vi "Motion Compensation Metrics.vi"() -> ()   [LabVIEW 2011]
uses:
  <vilib>/vision/NI_Vision_Development_Module.lvlib
panel:
  out "Waveform Chart 6":sgl(graph)
  out "Waveform Chart 5":sgl(graph)
  out "Waveform Chart 4":sgl(graph)
  out "Waveform Chart 3":sgl(graph)
  out "Waveform Chart 2":sgl[](graph)
  out "Waveform Chart":sgl[](graph)
  # "Orginal"
  # "Stabilized"
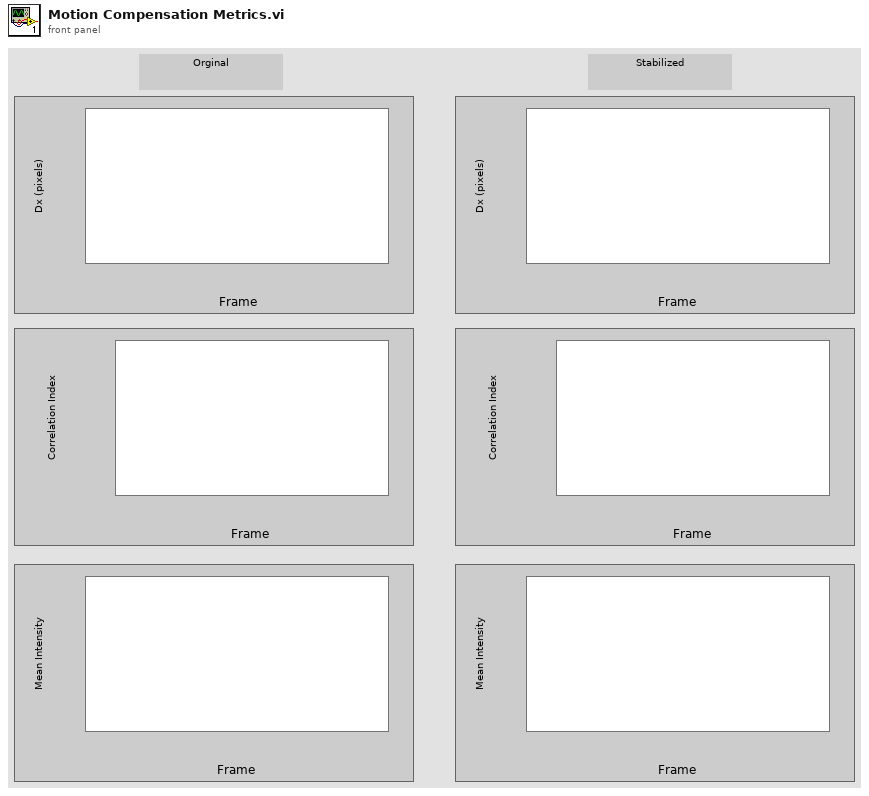
[diagram p1: front panel]
types:
  T1 = typedef "AviRefnum.ctl" = refnum<k1>
  T2 = typedef "IMAQ Image.ctl" = refnum<image>
  T3 = typedef "IMAQ Rectangle" = cluster{"Left":i32, "Top":i32, "Right":i32, "Bottom":i32, "Rotation":dbl}
  T4 = typedef "ROI Descriptor" = cluster{"Global Rectangle":i32[], "Contours":cluster{"ID":enum32{"External", "Internal"}, "Type":u32, "Coordinates":i32[]}[]}
  T5 = cluster{"Mean Intensity":sgl, "Standard  Deviation":sgl, "Minimum Intensity":sgl, "Maximum Intensity":sgl}
  T6 = cluster{"Position":cluster{"x":sgl, "y":sgl}, "Angle":sgl, "Scale":sgl, "Score":sgl, "Bounding Box":cluster{"x":sgl, "y":sgl}[]}[]
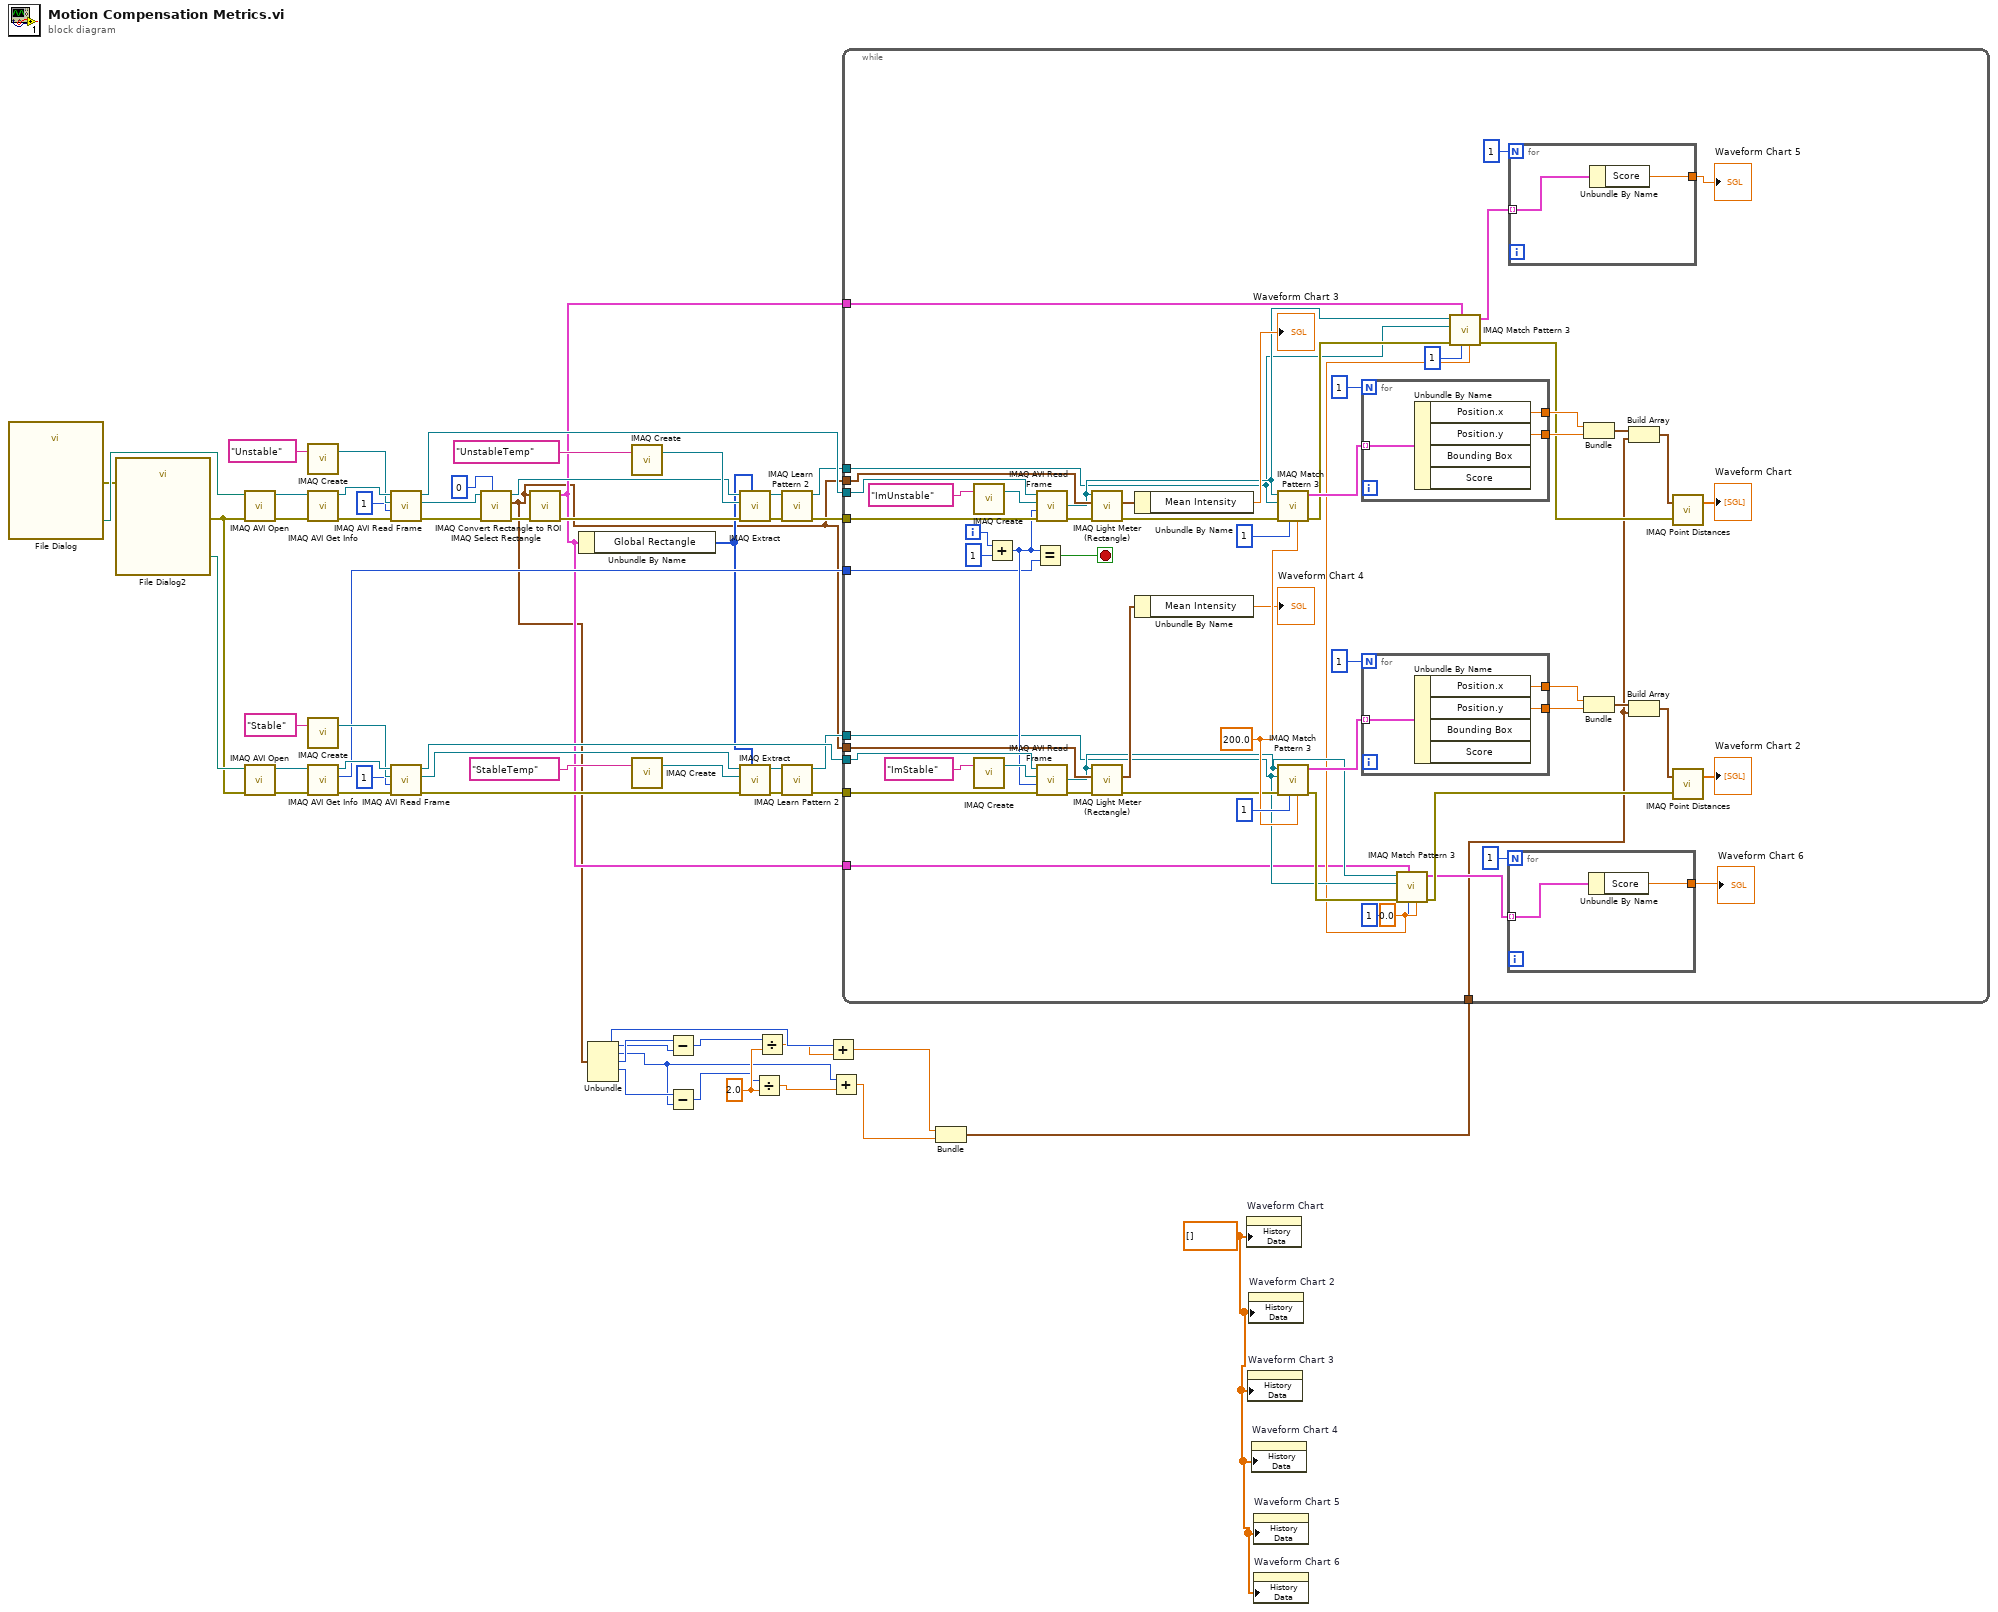
[diagram p0: block diagram]
diagram:
  w11 = 2.0 ("y")
  w14 = sgl[] [] ("History Data")
  n1 = call "File Dialog"() -> ("selected path"=w53:path, "error out"=w45:errorcluster)  [unwired: 12 in, 2 out]
  n2 = call "File Dialog2"("error in"=w45) -> ("selected path"=w52:path, "error out"=w44:errorcluster)  [unwired: 11 in, 2 out]
  n3 = call "IMAQ AVI Open"("error in (no error)"=w44, "AVI Path"=w53) -> ("error out"=w56:errorcluster, "Avi Refnum"=w51:T1)  [unwired: 8 in]
  n4 = call "IMAQ AVI Open"("error in (no error)"=w44, "AVI Path"=w52) -> ("error out"=w57:errorcluster, "Avi Refnum"=w50:T1)  [unwired: 8 in]
  n5 = call "IMAQ Create"("Image Name"="Unstable") -> ("New Image"=w46:T2)  [unwired: 4 in, 1 out]
  n6 = call "IMAQ AVI Get Info"("error in (no error)"=w56, "Avi Refnum"=w51) -> ("error out"=w55:errorcluster, "Avi Refnum (duplicate)"=w49:T1)  [unwired: 5 in, 3 out]
  n7 = call "IMAQ Create"("Image Name"="Stable") -> ("New Image"=w47:T2)  [unwired: 4 in, 1 out]
  n8 = call "IMAQ AVI Get Info"("error in (no error)"=w57, "Avi Refnum"=w50) -> ("error out"=w54:errorcluster, "Number of Frames"=w32:u32, "Avi Refnum (duplicate)"=w48:T1)  [unwired: 5 in, 2 out]
  n9 = call "IMAQ AVI Read Frame"("error in (no error)"=w55, "Frame Number"=u32 1, "Image"=w46, "Avi Refnum"=w49) -> ("error out"=w22:errorcluster, "Image Out"=w18:T2, "Avi Refnum (duplicate)"=w34:T1)  [unwired: 4 in, 1 out]
  n10 = call "IMAQ AVI Read Frame"("error in (no error)"=w54, "Frame Number"=u32 1, "Image"=w47, "Avi Refnum"=w48) -> ("error out"=w37:errorcluster, "Image Out"=w31:T2, "Avi Refnum (duplicate)"=w33:T1)  [unwired: 4 in, 1 out]
  n11 = call "IMAQ Select Rectangle"("Window Number (0...15)"=0, "error in (no error)"=w22, "Image In"=w18) -> ("error out"=w20:errorcluster, "Rectangle"=w12:T3, "Image Out (duplicate)"=w19:T2)  [unwired: 5 in, 1 out]
  n12 = call "IMAQ Convert Rectangle to ROI"("error in (no error)"=w20, "Rectangle"=w12) -> ("error out"=w17:errorcluster, "ROI Descriptor"=w15:T4)  [unwired: 7 in]
  n13 = Unbundle By Name(w15) -> ("Global Rectangle"=w16:i32[])
  n14 = Unbundle(w12) -> ("Left"=w6:i32, "Top"=w4:i32, "Right"=w10:i32, "Bottom"=w8:i32)  [unwired: 1 out]
  n15 = call "IMAQ Create"("Image Name"="UnstableTemp") -> ("New Image"=w41:T2)  [unwired: 4 in, 1 out]
  n16 = call "IMAQ Create"("Image Name"="StableTemp") -> ("New Image"=w40:T2)  [unwired: 4 in, 1 out]
  n17 = Subtract(x=w10, y=w6) -> (x-y=w9:i32)
  n18 = Subtract(x=w8, y=w4) -> (x-y=w7:i32)
  n19 = call "IMAQ Extract"("Optional Rectangle"=w16, "error in (no error)"=w17, "Image Dst"=w41, "Image Src"=w19) -> ("error out"=w30:errorcluster, "Image Dst Out"=w28:T2)  [unwired: 6 in]
  n20 = call "IMAQ Extract"("Optional Rectangle"=w16, "error in (no error)"=w37, "Image Dst"=w40, "Image Src"=w31) -> ("error out"=w26:errorcluster, "Image Dst Out"=w24:T2)  [unwired: 6 in]
  n21 = Divide(x=w7, y=w11) -> (x/y=w3:dbl)
  n22 = Divide(x=w9, y=w11) -> (x/y=w5:dbl)
  n23 = call "IMAQ Learn Pattern 2"("error in (no error)"=w30, "Image"=w28) -> ("error out"=w29:errorcluster, "Template Image Out"=w27:T2)  [unwired: 8 in]
  n24 = call "IMAQ Learn Pattern 2"("error in (no error)"=w26, "Image"=w24) -> ("error out"=w25:errorcluster, "Template Image Out"=w23:T2)  [unwired: 8 in]
  n25 = Add(x=w6, y=w5) -> (x+y=w2:dbl)
  n26 = Add(x=w4, y=w3) -> (x+y=w1:dbl)
  n27 = Bundle(w2, w1) -> (w13:cluster{dbl, dbl})  [unwired: 1 in]
  n28 = while {
    tunnel: w29 -> [w115]
    tunnel: w34 -> [w114]
    tunnel: w33 -> [w113]
    tunnel: w32 -> [w106]
    tunnel: w27 -> [w72]
    tunnel: w25 -> [w88]
    tunnel: w23 -> [w70]
    tunnel: w12 -> [w87]
    tunnel: w12 -> [w86]
    tunnel: w15 -> [w62]
    tunnel: w15 -> [w61]
    tunnel: w13 -> [w58]
    i -> [w117]
    stop <- w108 stop-if-true
    w69 = sgl 0.0 ("Minimum Match Score")
    w89 = sgl 200.0 ("Minimum Match Score")
    n29 = call "IMAQ Create"("Image Name"="ImUnstable") -> ("New Image"=w111:T2)  [unwired: 4 in, 1 out]
    n30 = call "IMAQ Create"("Image Name"="ImStable") -> ("New Image"=w112:T2)  [unwired: 4 in, 1 out]
    n31 = Add(x=w117, y=1) -> (x+y=w107:i32)
    n32 = Equal?(x=w107, y=w106) -> (x = y?=w108:bool)
    n33 = call "IMAQ AVI Read Frame"("error in (no error)"=w115, "Frame Number"=w107, "Image"=w111, "Avi Refnum"=w114) -> ("error out"=w85:errorcluster, "Image Out"=w73:T2)  [unwired: 4 in, 2 out]
    n34 = call "IMAQ AVI Read Frame"("error in (no error)"=w88, "Frame Number"=w107, "Image"=w112, "Avi Refnum"=w113) -> ("error out"=w83:errorcluster, "Image Out"=w71:T2)  [unwired: 4 in, 2 out]
    n35 = call "IMAQ Light Meter (Rectangle)"("error in (no error)"=w85, "Rectangle"=w87, "Image"=w73) -> ("error out"=w84:errorcluster, "Gray Level Intensities"=w81:T5)  [unwired: 4 in, 3 out]
    n36 = call "IMAQ Light Meter (Rectangle)"("error in (no error)"=w83, "Rectangle"=w86, "Image"=w71) -> ("error out"=w82:errorcluster, "Gray Level Intensities"=w79:T5)  [unwired: 4 in, 3 out]
    n37 = Unbundle By Name(w81) -> ("Mean Intensity"=→"Waveform Chart 3":sgl)
    n38 = Unbundle By Name(w79) -> ("Mean Intensity"=→"Waveform Chart 4":sgl)
    n39 = call "IMAQ Match Pattern 3"("Minimum Match Score"=w89, "Number of Matches Requested"=1, "error in (no error)"=w84, "Template Image"=w72, "Image"=w73) -> ("error out"=w75:errorcluster, "Matches"=w101:T6)  [unwired: 4 in, 1 out]
    n40 = call "IMAQ Match Pattern 3"("Minimum Match Score"=w89, "Number of Matches Requested"=1, "error in (no error)"=w82, "Template Image"=w70, "Image"=w71) -> ("error out"=w77:errorcluster, "Matches"=w100:T6)  [unwired: 4 in, 1 out]
    n41 = for {
      N: 1 -> [_]
      tunnel: w101 -> [w127] mode=indexing
      tunnel: [w126] -> w99
      tunnel: [w125] -> w98
      n42 = Unbundle By Name(w127) -> ("Position.x"=w126:sgl, "Position.y"=w125:sgl)  [unwired: 2 out]
    }
    n43 = for {
      N: 1 -> [_]
      tunnel: w100 -> [w124] mode=indexing
      tunnel: [w123] -> w97
      tunnel: [w122] -> w96
      n44 = Unbundle By Name(w124) -> ("Position.x"=w123:sgl, "Position.y"=w122:sgl)  [unwired: 2 out]
    }
    n45 = call "IMAQ Match Pattern 3"("Minimum Match Score"=w69, "Number of Matches Requested"=1, "ROI Descriptor"=w61, "error in (no error)"=w77, "Template Image"=w70, "Image"=w71) -> ("error out"=w76:errorcluster, "Matches"=w66:T6)  [unwired: 3 in, 1 out]
    n46 = call "IMAQ Match Pattern 3"("Minimum Match Score"=w69, "Number of Matches Requested"=1, "ROI Descriptor"=w62, "error in (no error)"=w75, "Template Image"=w72, "Image"=w73) -> ("error out"=w74:errorcluster, "Matches"=w64:T6)  [unwired: 3 in, 1 out]
    n47 = for {
      N: 1 -> [_]
      tunnel: w66 -> [w119] mode=indexing
      tunnel: [w118] -> w59
      n48 = Unbundle By Name(w119) -> ("Score"=w118:sgl)
    }
    "Waveform Chart 6" <- w59
    n49 = for {
      N: 1 -> [_]
      tunnel: [w121] -> w60
      tunnel: w64 -> [w120] mode=indexing
      n50 = Unbundle By Name(w120) -> ("Score"=w121:sgl)
    }
    "Waveform Chart 5" <- w60
    n51 = Bundle("x"=w99, "y"=w98) -> (w95:cluster{"x":sgl, "y":sgl})  [unwired: 1 in]
    n52 = Bundle("x"=w97, "y"=w96) -> (w93:cluster{"x":sgl, "y":sgl})  [unwired: 1 in]
    n53 = Build Array(w95, w58) -> (w94:cluster{"x":dbl, "y":dbl}[])
    n54 = Build Array(w93, w58) -> (w92:cluster{"x":dbl, "y":dbl}[])
    n55 = call "IMAQ Point Distances"("Points"=w94, "error in (no error)"=w74) -> ("Distances"=→"Waveform Chart":sgl[])  [unwired: 3 in, 1 out]
    n56 = call "IMAQ Point Distances"("Points"=w92, "error in (no error)"=w76) -> ("Distances"=→"Waveform Chart 2":sgl[])  [unwired: 3 in, 1 out]
  }
  n57 = property on="Waveform Chart" class="WFChart (strict)"("History Data"=w14) -> ()  [unwired: 2 in, 2 out]
  n58 = property on="Waveform Chart 3" class="WFChart (strict)"("History Data"=w14) -> ()  [unwired: 2 in, 2 out]
  n59 = property on="Waveform Chart 2" class="WFChart (strict)"("History Data"=w14) -> ()  [unwired: 2 in, 2 out]
  n60 = property on="Waveform Chart 4" class="WFChart (strict)"("History Data"=w14) -> ()  [unwired: 2 in, 2 out]
  n61 = property on="Waveform Chart 5" class="WFChart (strict)"("History Data"=w14) -> ()  [unwired: 2 in, 2 out]
  n62 = property on="Waveform Chart 6" class="WFChart (strict)"("History Data"=w14) -> ()  [unwired: 2 in, 2 out]
